vi "Do.vi"(8 "error in (no error)":errorcluster, 10 "Actor in":refnum<class "Actor.lvclass">, 11 "Addition Request Msg":refnum<class "Addition Request Msg.lvclass">) -> (0 "error out":errorcluster, 2 "Actor out":refnum<class "Actor.lvclass">)   [LabVIEW 2015, in "Addition Request Msg.lvclass"]
doc: "(<B>Filename</B>: Actor Framework.lvlib:Message.lvclass:Do.vi)\n\nDefines what a message does when it is received by an actor. Generally, a message instructs an actor to invoke one of its methods. By default, this method does nothing. A child class must override it to define behavior. Create a child class by using the Actor Framework Message Maker dialog box."
uses:
  Addition Request Msg.lvclass
  <vilib>/ActorFramework/Actor/Actor.lvclass
  Addition Actor Class/Addition Actor.lvclass
  Addition Request Msg.lvclass/Addition Request Msg.ctl
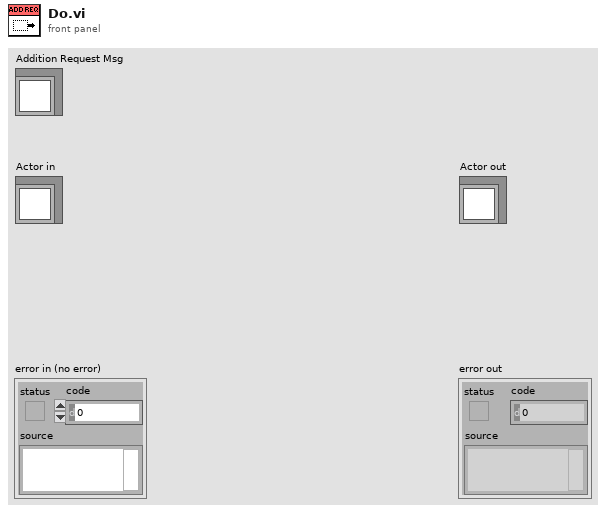
[diagram p1: front panel]
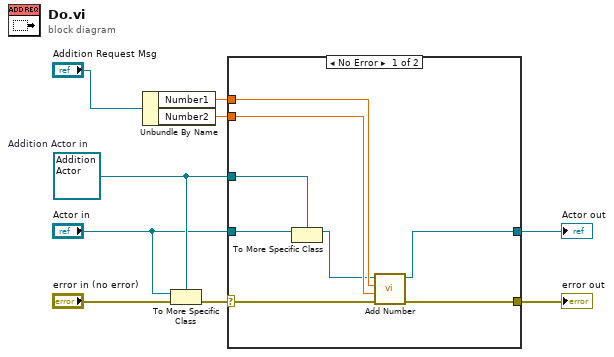
[diagram p0: block diagram]
diagram:
  w2 = refnum<class "Addition Actor.lvclass"> refnum  # Addition Actor in
  n1 = Unbundle By Name("Addition Request Msg") -> ("Number1"=w5:dbl, "Number2"=w4:dbl)
  n2 = To More Specific Class(target class=w2, reference="Actor in", error in="error in (no error)") -> (error out=w8:errorcluster)  [unwired: 1 out]
  n3 = case shown="No Error" w8 {
    selector: w8 -> [w16 w18]
    tunnel: "Actor in" -> [w17 w19]
    tunnel: [w15 w18] -> w7
    tunnel: w5 -> [w14 _]
    tunnel: w4 -> [w13 _]
    tunnel: w2 -> [w12 _]
    tunnel: [w10 w19] -> w3
    frame No Error {
      n4 = To More Specific Class(target class=w12, reference=w17) -> (specific class reference=w11:refnum<class "Addition Actor.lvclass">)  [unwired: 1 in, 1 out]
      n5 = call "Add Number.vi"("error in (no error)"=w16, "Number2"=w13, "Number1"=w14, "Addition Actor in"=w11) -> ("error out"=w15:errorcluster, "Addition Actor out"=w10:refnum<class "Addition Actor.lvclass">)  [unwired: 6 in]
    }
    frame Error {
    }
  }
  "error out" <- w7
  "Actor out" <- w3
